vi "RgbaToU64_2D.vi"(11 "Rgba":T1[][](array[typedef])) -> (3 "U64":u64[][](array[numeric]))   [LabVIEW 2024, in "OpenLvVision_Image.lvlib" / "DataAccess.lvlib"]
doc: "Convert an color cluster into an number"
uses:
  DataAccess.lvlib
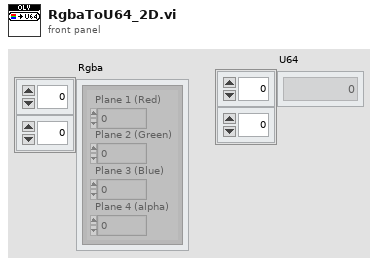
[diagram p1: front panel]
types:
  T1 = typedef "Color (U64)" = cluster{"Plane 3 (Blue)":u16, "Plane 2 (Green)":u16, "Plane 1 (Red)":u16, "Plane 4 (alpha)":u16}
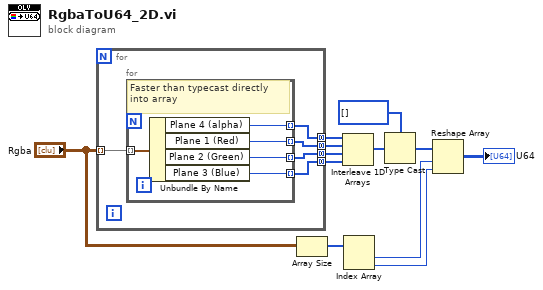
[diagram p0: block diagram]
diagram:
  n1 = for {
    tunnel: [w17] -> w12 mode=concatenating
    tunnel: [w16] -> w11 mode=concatenating
    tunnel: [w15] -> w10 mode=concatenating
    tunnel: [w14] -> w9 mode=concatenating
    tunnel: "Rgba" -> [w13] mode=indexing
    n2 = for {
      tunnel: [w22] -> w17 mode=indexing
      tunnel: [w21] -> w15 mode=indexing
      tunnel: [w20] -> w16 mode=indexing
      tunnel: [w19] -> w14 mode=indexing
      tunnel: w13 -> [w18] mode=indexing
      # "Faster than typecast directly into array"
      n3 = Unbundle By Name(w18) -> ("Plane 4 (alpha)"=w22:u16, "Plane 1 (Red)"=w21:u16, "Plane 2 (Green)"=w20:u16, "Plane 3 (Blue)"=w19:u16)
    }
  }
  n4 = Array Size(array="Rgba") -> (size(s)=w5:i32[])
  n5 = Interleave 1D Arrays(w12, w10, w11, w9) -> (w8:u16[])
  n6 = Index Array(array=w5) -> (element #1=w4:i32, element #2=w3:i32)  [unwired: 2 in]
  n7 = Type Cast(type=u64[] [], x=w8) -> (*(type *) &x=w6:u64[])
  n8 = Reshape Array(w6, w4, w3) -> (→"U64":u64[][])
